vi "arrow_keys_demo.vi"() -> ()   [LabVIEW 2009]
panel:
  in  "stop":bool
  # "Run VI and then press arrow keys .\nLet me know on the message boards if you have any questions\n-Steve"
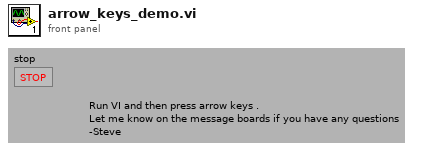
[diagram p1: front panel]
types:
  T1 = typedef "eventvkey.ctl" = enum16{"ASCII", "Enter", "Return", "Shift", "Ctrl", "Alt", "Cmd", "Opt", "Caps", "NumLock", "Clear", "Break", "Up", "Down", "Left", "Right", "Insert", "Delete", "Home", "End", "PageUp", "PageDown", "Escape", "Help", "Pause", "ScrollLock", "F1", "F2", "F3", "F4", "F5", "F6", "F7", "F8", "F9", "F10", "F11", "F12", "F13", "F14", "F15", "F16", "F17", "F18", "F19", "F20", "F21", "F22", "F23", "F24", "Play", "VolumeUp", "VolumeDown", "Mute", "Two Byte Char"}
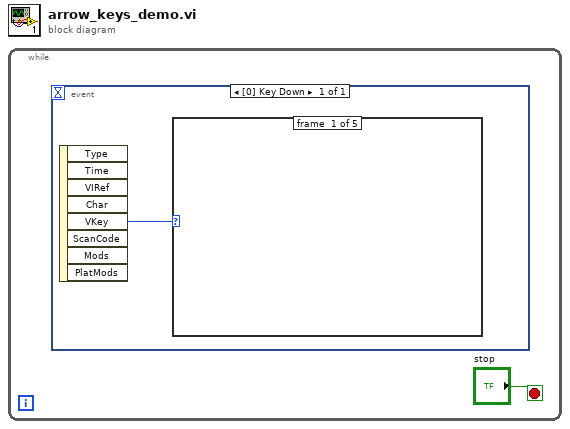
[diagram p0: block diagram]
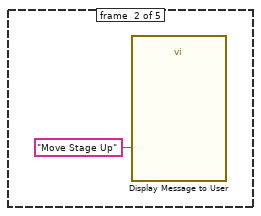
[diagram p2: hidden frame]
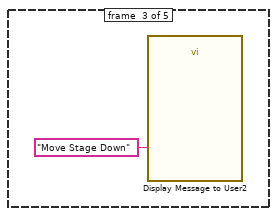
[diagram p3: hidden frame]
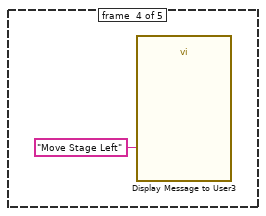
[diagram p4: hidden frame]
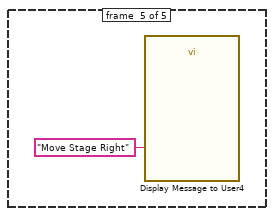
[diagram p5: hidden frame]
diagram:
  n1 = while {
    stop <- "stop" stop-if-true
    n2 = event shown="[0] Key Down" {
      selector: _ -> [_]
      dyn-events: _ -> [_]
      timeout: _ -> [_]
      event [0] Key Down {
        n3 = event-data() -> ("VKey"=w2:T1)  [unwired: 1 in, 7 out]
        n4 = case shown="\"Up\"" w2 {
          frame #0 {
          }
          frame #1 {
            n5 = call "Display Message to User"("Message"="Move Stage Up") -> ()  [unwired: 9 in, 2 out]
          }
          frame #2 {
            n6 = call "Display Message to User2"("Message"="Move Stage Down") -> ()  [unwired: 9 in, 2 out]
          }
          frame #3 {
            n7 = call "Display Message to User3"("Message"="Move Stage Left") -> ()  [unwired: 9 in, 2 out]
          }
          frame #4 {
            n8 = call "Display Message to User4"("Message"="Move Stage Right") -> ()  [unwired: 9 in, 2 out]
          }
        }
      }
    }
  }
